vi "KI6221.vi"() -> ()   [LabVIEW 2025] (continued)
                        n2236 = Number To Engineering String(4:w3702) -> (0:w3710:string)  [unwired: 3 in]
                        n2237 = Number To Engineering String(4:w3694) -> (0:w3709:string)  [unwired: 3 in]
                        n2238 = Number To Engineering String(4:w3701) -> (0:w3723:string)  [unwired: 3 in]
                        n2239 = Number To Engineering String(4:w3722) -> (0:w3721:string)  [unwired: 3 in]
                        n2240 = Absolute Value(x=w3701) -> (abs(x)=w3719:dbl)
                        n2241 = Absolute Value(x=w3702) -> (abs(x)=w3720:dbl)
                        n2242 = local read "DAMPING"() -> (w3707:bool)
                        n2243 = local read "Voltage Measure Range"() -> (w3703:dbl)
                        n2244 = Greater?(x=w3719, y=w3720) -> (0:w3717:bool)
                        n2245 = Select(t=w3719, s=w3717, f=w3720) -> (s? t:f=w3718:dbl)
                        n2246 = Number To Exponential String(number=w3718) -> (E-format string=w3705:string)  [unwired: 3 in]
                        n2247 = Boolean To (0,1)(Boolean=w3707) -> (0, 1=w3708:i16)
                        n2248 = Number To Decimal String(number=w3700) -> (decimal integer string=w3714:string)  [unwired: 1 in]
                        n2249 = Number To Exponential String(number=w3703) -> (E-format string=w3704:string)  [unwired: 3 in]
                        n2250 = Number To Decimal String(number=w3708) -> (decimal integer string=w3706:string)  [unwired: 1 in]
                        n2251 = case shown="1" w3699 {
                          tunnel: w3714 -> [w3732 w3736 w3739]
                          tunnel: [w3732 w3736 w3739] -> w3711
                          tunnel: ["MOV" "MOV" "REP"] -> w3713
                          tunnel: ["0" "1" "1"] -> w3712
                          frame 0, Default {
                          }
                          frame 1 {
                          }
                          frame 2 {
                          }
                        }
                        n2252 = Insert Into Array(array=string[] [], new element #1=w3724, new element #2=w3723, new element #3=w3721, new element #4=w3704, new element #5=w3715, new element #6=w3713, new element #7=w3712, new element #8=w3711, new element #9=w3710, new element #10=w3709, new element #11=w3706, new element #12=w3705) -> (w3726:string[])  [unwired: 1 in]
                        n2253 = call "VisaVarReplace.vi"("Replace Array"=w3726, "Search Array"=string[] ["<DEMOSETUPSTRING>", "<DEMOSOURCE>", "<DEMOCOMP>", "<DEMORANGE>", "<DEMODELTANPLC>", "<DEMOFTYPE>", "<DEMOFSTATE>", "<DEMOFCOUNT>", "<DELTALOW>", "<DELTADELAY>", "<DELTADAMPING>", "<DELTACURRRANGE>"], "GPIB Array"=w3729) -> ("GPIB Array OUT"=w3728:string[])
                        n2254 = call "DeltaModeDemo.vi"("6220 VISA Ref"=w3730, "GPIB ARRAY"=w3728, "Current HI"=w3698, "Current LO"=w3697) -> ()  [unwired: 12 in]
                      }
                    }
                  }
                }
                n2255 = case shown="True" "CLEAR DELTA DATA" {
                  frame False {
                  }
                  frame True {
                    n2256 = invoke on="Delta Mode Measurement Data" class="Table" method="Reinit To Default"() -> ()  [unwired: 3 in, 3 out]
                    n2257 = invoke on="Delta Mode Resistance Graph" class="XYGraph (strict)" method="Reinit To Default"() -> ()  [unwired: 3 in, 3 out]
                  }
                }
                n2258 = case shown="1, Default" "FILTER" {
                  tunnel: [FALSE TRUE] -> w3669
                  frame 0 {
                  }
                  frame 1, Default {
                  }
                }
                n2259 = property on="Filter\nCount" class="DigNum (strict)"("Visible"=w3669) -> ()  [unwired: 2 in, 2 out]
                n2260 = case shown="True" "SAVE DELTA DATA" {
                  frame False {
                  }
                  frame True {
                    n2261 = File Dialog(4:"KI Data files" ("pattern label"), 5:"Save As" ("button label"), 6:"*.kdf" ("pattern label")) -> (1:w4176:bool, 3:w4175:path)  [unwired: 4 in, 2 out]
                    n2262 = case shown="False" w4176 {
                      tunnel: w4175 -> [w4180 _]
                      frame False {
                        w4184 = "%s" ("format string")
                        n2263 = property on="Delta Mode Measurement Data" class="Tbl (strict)"() -> ("Column Header Strings[]"=w4185:string[], "Value"=w4186:string[][])  [unwired: 2 in, 2 out]
                        n2264 = Array To Spreadsheet String(array=w4186, 3:w4184) -> (spreadsheet string=w4182:string)  [unwired: 1 in]
                        n2265 = Array To Spreadsheet String(array=w4185, 3:w4184) -> (spreadsheet string=w4183:string)  [unwired: 1 in]
                        n2266 = Concatenate Strings(w4183, w4182) -> (w4181:string)
                        n2267 = call "WriteToFile.vi"("character string"=w4181, "file path (dialog if empty)"=w4180) -> ()  [unwired: 3 in, 1 out]
                      }
                      frame True {
                      }
                    }
                  }
                }
                n2268 = Boolean To (0,1)(Boolean="INFINITE DELTA CYCLES") -> (0, 1=w3667:i16)
                n2269 = Multiply(x=w3667, y=i16 2) -> (x*y=w3666:i16)
                n2270 = property on="Number of cycles" class="DigNum (strict)"("Disabled"=w3666) -> ()  [unwired: 2 in, 2 out]
                n2271 = local read "Delta Mode Measurement Data"() -> (w3649:string[][])
                n2272 = local read "X AXIS LAST -DELTA"() -> (w3647:i32)
                n2273 = local read "Y AXIS LAST -DELTA"() -> (w3646:i32)
                n2274 = property on="X Axis:" class="Ring (strict)"() -> ("Value"=w3659:u16, "Strings []"=w3657:string[])  [unwired: 2 in, 2 out]
                n2275 = property on="Y Axis:" class="Ring (strict)"() -> ("Value"=w3658:u16, "Strings []"=w3656:string[])  [unwired: 2 in, 2 out]
                n2276 = Array Size(array=w3649) -> (size(s)=w3655:i32[])
                n2277 = Equal?(x=w3646, y=w3658) -> (x = y?=w3662:bool)
                n2278 = Index Array(array=w3655) -> (element=w3653:i32)  [unwired: 1 in]
                n2279 = Index Array(array=w3655) -> (element=w3654:i32)  [unwired: 1 in]
                n2280 = Equal?(x=w3647, y=w3659) -> (x = y?=w3661:bool)
                n2281 = And(x=w3661, y=w3662) -> (x .and. y?=w3660:bool)
                n2282 = Add(x=w3654, y=w3653) -> (x+y=w3652:i32)
                n2283 = Equal To 0?(x=w3652) -> (x = 0?=w3650:bool)
                n2284 = Or(x=w3660, y=w3650) -> (x .or. y?=w3651:bool)
                n2285 = case shown="False" w3651 {
                  tunnel: w3659 -> [w3741 _]
                  tunnel: w3658 -> [w3742 _]
                  tunnel: w3657 -> [w3747 _]
                  tunnel: w3656 -> [w3746 _]
                  tunnel: w3649 -> [w3743 _]
                  frame False {
                    n2286 = Index Array(array=w3747, index=w3741) -> (element=w3745:string)
                    n2287 = Index Array(array=w3746, index=w3742) -> (element=w3744:string)
                    n2288 = Add(x=w3742, y=2) -> (x+y=w3748:i32)
                    n2289 = property on="Delta Mode Resistance Graph" class="XYGraph (strict)"("X Scale.Name Label.Text"=w3745, "Y Scale.Name Label.Text"=w3744) -> ()  [unwired: 2 in, 2 out]
                    n2290 = Index Array(array=w3743, index (col)=w3741) -> (element=w3754:string[])  [unwired: 1 in]
                    n2291 = Index Array(array=w3743, index (col)=w3748) -> (element=w3751:string[])  [unwired: 1 in]
                    n2292 = Fract/Exp String To Number(string=w3754) -> (number=w3753:dbl[])  [unwired: 3 in, 1 out]
                    n2293 = Fract/Exp String To Number(string=w3751) -> (number=w3750:dbl[])  [unwired: 3 in, 1 out]
                    n2294 = call "Convert to Dynamic Data7"("Array"=w3753) -> ("Dynamic Data Type"=w3752:dynamicdata)  [unwired: 3 in]
                    n2295 = call "Convert to Dynamic Data8"("Array"=w3750) -> ("Dynamic Data Type"=w3749:dynamicdata)  [unwired: 3 in]
                    n2296 = call "Build XY Graph5"("Y Input"=w3749, "X Input"=w3752) -> ("XY Graph"=→"Delta Mode Resistance Graph":cluster{"Y":dbl[], "Y":dbl[]}[])  [unwired: 8 in, 1 out]
                    "Y AXIS LAST -DELTA" <- w3742
                    "X AXIS LAST -DELTA" <- w3741
                  }
                  frame True {
                  }
                }
              }
              frame "ARB Waveform Generator" {
                # "TURNS OFF SCALAR WHEN ITEM IS SELECTED IN CALC WINDOW 2"
                # "This inserts waves selected on\n the scratchpad into the \nComplete waveform."
                # "This deletes the highlighted \nwave from the scratchpad."
                # "ADD to the SCRATCHPAD. Whenever possible Labview signal generator subvis are used. \nElse they the signal is created in while loops."
                # "This saves the complete wave to a TEXT FILE."
                # "Updates the GRAPH\npreview based on \nthe view and \nselection settings."
                # "Update enable state based \non checkbox."
                # "Updates the tabs to match \nthe RING."
                # "These below are the segments for the GUI response to changes in the RING & Checkbox Controls."
                # "This section runs the ARB upload, run, and stop buttons. This \nsends all the information to the instrument for these buttons."
                # "Takes a complete wave and compacts it into\none wave on the scratchpad."
                # "These are controls referenced, but not directly used\nin the ARB."
                # "This is the option in the case statement for the ARB Waveform Generator. The buttons are attached to case statements that function only when the button is pressed."
                # "PHASE SETUP window. Sets the state, triggerline, and angle \n                                for the Phase marker."
                n2297 = Equal?(x=u16 4, y="Waveform Type") -> (x = y?=w4202:bool)
                n2298 = Equal?(x="Custom points file:", y=path "") -> (x = y?=w4203:bool)
                n2299 = And(x=w4203, y=w4202) -> (x .and. y?=w4199:bool)
                n2300 = Not(x=w4199) -> (.not. x?=w4198:bool)
                n2301 = And(x="ADD SCRATCH", y=w4198) -> (x .and. y?=w4200:bool)
                n2302 = case shown="True" "<- Compact" {
                  tunnel: "waveform holder" -> [_ w4280]
                  frame False {
                  }
                  frame True {
                    n2303 = control-ref of="ScratchPad"() -> (w4288:refnum<vi>)
                    n2304 = control-ref of="Complete Waveform"() -> (w4284:refnum<vi>)
                    n2305 = control-ref of="ADD"() -> (w4283:refnum<vi>)
                    n2306 = control-ref of="ADD 2"() -> (w4282:refnum<vi>)
                    n2307 = control-ref of="filter"() -> (w4281:refnum<vi>)
                    n2308 = control-ref of="ScratchPad Array"() -> (w4287:refnum<vi>)
                    n2309 = control-ref of="ScratchPad Array Cnt"() -> (w4286:refnum<vi>)
                    n2310 = control-ref of="empty"() -> (w4285:refnum<vi>)
                    n2311 = call "WaveCompact.vi"("reference"=w4288, "waveform holder"=w4280, "reference 2"=w4287, "reference 3"=w4286, "reference 5"=w4284, "reference 4"=w4285, "reference 8"=w4281, "reference 7"=w4282, "reference 6"=w4283) -> ()
                  }
                }
                n2312 = case shown="True" "Save to File" {
                  tunnel: "waveform holder" -> [_ w4297]
                  frame False {
                  }
                  frame True {
                    n2313 = property on="Complete Waveform" class="LstBox (strict)"() -> ("Item Names"=w4301:string[])  [unwired: 2 in, 2 out]
                    n2314 = Index Array(array=w4301, index=0) -> (element=w4300:string)
                    n2315 = Equal?(x=w4300, y="") -> (x = y?=w4298:bool)
                    n2316 = case shown="False" w4298 {
                      tunnel: w4297 -> [w4305 _]
                      frame False {
                        n2317 = File Dialog(4:"data.txt", 6:"*.txt") -> (1:w4307:bool, 3:w4306:path)  [unwired: 5 in, 2 out]
                        n2318 = case shown="False" w4307 {
                          tunnel: w4305 -> [w4311 _]
                          tunnel: w4306 -> [w4309 _]
                          frame False {
                            n2319 = call-poly <vilib>:"Write To Spreadsheet File.vi"("transpose? (no:F)"=TRUE, "format (%.3f)"="%.6e", "1D data"=w4311, "file path (dialog if empty)"=w4309) -> ()  [unwired: 4 in, 1 out]
                          }
                          frame True {
                          }
                        }
                      }
                      frame True {
                        n2320 = call "Display Message to User17"() -> ()  [unwired: 10 in, 2 out]
                      }
                    }
                  }
                }
                n2321 = case shown="True" w4200 {
                  tunnel: "Waveform Type" -> [_ w4367]
                  tunnel: "Custom points file:" -> [_ w4369]
                  frame False {
                  }
                  frame True {
                    n2322 = Increment(x="Rise/Fall in points") -> (x+1=w4335:i32)
                    n2323 = property on="ADD SCRATCH" class="Bool"("Disabled"=2 ("index")) -> (error out=w4340:errorcluster)  [unwired: 2 in, 1 out]
                    n2324 = property on="ScratchPad" class="LstBox (strict)"() -> ("Item Names"=w4374:string[])  [unwired: 2 in, 2 out]
                    n2325 = call "WaveErrorFlags.vi"("Rise/Fall in points"=w4335, "Number of Points per cycle"="Number of Points per cycle", "Waveform Type"=w4367, "Item Names"=w4374) -> ("Boolean 2"=w4371:bool, "Boolean 5"=w4375:bool, "Boolean 4"=w4373:bool, "Boolean"=w4370:bool, "Boolean 3"=w4372:bool)
                    n2326 = case shown="False" w4375 {
                      tunnel: w4373 -> [_ w4495]
                      tunnel: w4372 -> [_ w4494]
                      tunnel: w4371 -> [_ w4493]
                      tunnel: w4370 -> [_ w4492]
                      tunnel: w4369 -> [w4416 _]
                      tunnel: w4367 -> [w4415 _]
                      tunnel: "Analog filter - \nTau in # points" -> [w4414 _]
                      tunnel: "ADD" -> [w4413 _]
                      tunnel: "math" -> [w4412 _]
                      tunnel: "ADD 2" -> [w4411 _]
                      tunnel: "Number of Points per cycle" -> [w4410 _]
                      tunnel: "Number of Cycles" -> [w4409 _]
                      tunnel: "Standard Deviation" -> [w4408 _]
                      tunnel: "Offset (Amps)" -> [w4407 _]
                      tunnel: "Number of Points per cycle" -> [w4406 _]
                      tunnel: "Number of Cycles" -> [w4405 _]
                      tunnel: "Amplitude (Amps)" -> [w4404 _]
                      tunnel: "Offset (Amps)" -> [w4403 _]
                      tunnel: "Start Phase \n(Degrees)" -> [w4402 _]
                      tunnel: w4335 -> [w4401 _]
                      tunnel: "Number of Points per cycle" -> [w4400 _]
                      tunnel: "Number of Cycles" -> [w4399 _]
                      tunnel: "Amplitude (Amps)" -> [w4398 _]
                      tunnel: "Offset (Amps)" -> [w4397 _]
                      tunnel: "Start Phase \n(Degrees)" -> [w4396 _]
                      tunnel: "Duty Cycle (%)" -> [w4395 _]
                      tunnel: "Ramp to: (Amps)" -> [w4394 _]
                      tunnel: "Ramp from: (Amps)" -> [w4393 _]
                      tunnel: "Duty Cycle (%)" -> [w4392 _]
                      tunnel: "Start Phase \n(Degrees)" -> [w4391 _]
                      tunnel: "Number of Points per cycle" -> [w4390 _]
                      tunnel: "Number of Cycles" -> [w4389 _]
                      tunnel: w4340 -> [w4388 w4491]
                      tunnel: [w4388 w4491] -> w4338
                      tunnel: "Scalar?" -> [w4377 _]
                      tunnel: "Constant" -> [w4376 _]
                      frame False {
                        n2327 = property on="ScratchPad Array" class="Arr (strict)"() -> ("Value"=w4417:dbl[][])  [unwired: 2 in, 2 out]
                        n2328 = property on="ScratchPad Array Cnt" class="Arr (strict)"() -> ("Value"=w4418:i32[])  [unwired: 2 in, 2 out]
                        n2329 = property on="empty" class="Arr (strict)"() -> ("Value"=w4420:dbl[])  [unwired: 2 in, 2 out]
                        n2330 = case shown="1" w4415 {
                          tunnel: [w4429 w4441 w4451 w4460 w4466 w4476 w4484] -> w4422
                          tunnel: [w4433 w4444 w4454 w4463 w4470 w4477 w4486] -> w4419
                          tunnel: [w4432 w4445 w4455 w4464 errorcluster {"status"=FALSE, "code"=0, "source"=""} ("error out 9") errorcluster {"status"=FALSE, "code"=0, "source"=""} errorcluster {"status"=FALSE, "code"=0, "source"=""}] -> w4378
                          tunnel: [w4431 w4443 w4453 w4462 w4468 w4478 w4483] -> w4421
                          tunnel: w4420 -> [w4430 w4442 w4452 w4461 w4467 _ _]
                          tunnel: w4418 -> [_ _ _ _ _ w4480 w4489]
                          tunnel: w4417 -> [_ _ _ _ _ w4481 w4488]
                          tunnel: w4416 -> [_ _ _ _ w4465 _ _]
                          tunnel: w4414 -> [_ _ _ _ _ _ w4482]
                          tunnel: w4413 -> [_ _ _ _ _ w4475 _]
                          tunnel: w4412 -> [_ _ _ _ _ w4474 _]
                          tunnel: w4411 -> [_ _ _ _ _ w4473 _]
                          tunnel: w4410 -> [_ _ _ w4459 _ _ _]
                          tunnel: w4409 -> [_ _ _ w4458 _ _ _]
                          tunnel: w4408 -> [_ _ _ w4457 _ _ _]
                          tunnel: w4407 -> [_ _ _ w4456 _ _ _]
                          tunnel: w4406 -> [_ _ w4450 _ _ _ _]
                          tunnel: w4405 -> [_ _ w4449 _ _ _ _]
                          tunnel: w4404 -> [_ _ w4448 _ _ _ _]
                          tunnel: w4403 -> [_ _ w4447 _ _ _ _]
                          tunnel: w4402 -> [_ _ w4446 _ _ _ _]
                          tunnel: w4401 -> [_ w4440 _ _ _ _ _]
                          tunnel: w4400 -> [_ w4439 _ _ _ _ _]
                          tunnel: w4399 -> [_ w4438 _ _ _ _ _]
                          tunnel: w4398 -> [_ w4437 _ _ _ _ _]
                          tunnel: w4397 -> [_ w4436 _ _ _ _ _]
                          tunnel: w4396 -> [_ w4435 _ _ _ _ _]
                          tunnel: w4395 -> [_ w4434 _ _ _ _ _]
                          tunnel: w4394 -> [w4428 _ _ _ _ _ _]
                          tunnel: w4393 -> [w4427 _ _ _ _ _ _]
                          tunnel: w4392 -> [w4426 _ _ _ _ _ _]
                          tunnel: w4391 -> [w4425 _ _ _ _ _ _]
                          tunnel: w4390 -> [w4424 _ _ _ _ _ _]
                          tunnel: w4389 -> [w4423 _ _ _ _ _ _]
                          tunnel: w4377 -> [_ _ _ _ _ w4472 _]
                          tunnel: w4376 -> [_ _ _ _ _ w4471 _]
                          frame 0, Default {
                            n2331 = call "RampGen.vi"("Value 2"=w4430, "Ramp to: (Amps)"=w4428, "Ramp from: (Amps)"=w4427, "Number of Cycles"=w4423, "Duty Cycle (%)"=w4426, "Number of Points per cycle"=w4424, "Start Phase \n(Degrees)"=w4425) -> ("error"=w4432:errorcluster, "Numeric"=w4431:dbl, "String"=w4433:string, "Value"=w4429:dbl[])
                          }
                          frame 1 {
                            n2332 = call "SquareGen.vi"("Amplitude (Amps)"=w4437, "Number of Points per cycle"=w4439, "Number of Cycles"=w4438, "Value 2"=w4442, "Duty Cycle (%)"=w4434, "Offset (Amps)"=w4436, "Rise/Fall in points"=w4440, "Start Phase \n(Degrees)"=w4435) -> ("error"=w4445:errorcluster, "Numeric"=w4443:dbl, "String"=w4444:string, "Value"=w4441:dbl[])
                          }
                          frame 2 {
                            n2333 = call "SineGen.vi"("Start Phase \n(Degrees)"=w4446, "Value 2"=w4452, "Offset (Amps)"=w4447, "Amplitude (Amps)"=w4448, "Number of Points per cycle"=w4450, "Number of Cycles"=w4449) -> ("error"=w4455:errorcluster, "Numeric"=w4453:dbl, "String"=w4454:string, "Value"=w4451:dbl[])
                          }
                          frame 3 {
                            n2334 = call "NoiseGen.vi"("Offset (Amps)"=w4456, "Number of Cycles"=w4458, "Standard Deviation"=w4457, "Number of Points per cycle"=w4459, "Value 2"=w4461) -> ("error out 9"=w4464:errorcluster, "Numeric"=w4462:dbl, "String"=w4463:string, "Value"=w4460:dbl[])
                          }
                          frame 4 {
                            n2335 = call "CustomGen.vi"("Custom points file:"=w4465, "Value 2"=w4467) -> ("Value"=w4466:dbl[], "source"=w4470:string, "Numeric"=w4468:dbl)
                          }
                          frame 5 {
                            n2336 = call "CalcGen.vi"("Constant"=w4471, "Scalar?"=w4472, "Value 2"=w4480, "Value 3"=w4481, "ADD 2"=w4473, "ADD"=w4475, "math"=w4474) -> ("Numeric"=w4478:dbl, "source"=w4477:string, "Value"=w4476:dbl[])
                          }
                          frame 6 {
                            n2337 = call "FilterGen.vi"("SP ARRAY"=w4488, "Analog filter - \nTau in # points"=w4482, "Value 3"=w4489, "filter"="filter") -> ("Numeric"=w4483:dbl, "source"=w4486:string, "Value"=w4484:dbl[])
                          }
                        }
                        "error out 9" <- w4378
                        n2338 = control-ref of="ScratchPad"() -> (w4387:refnum<vi>)
                        n2339 = control-ref of="Complete Waveform"() -> (w4384:refnum<vi>)
                        n2340 = control-ref of="ADD"() -> (w4383:refnum<vi>)
                        n2341 = control-ref of="ADD 2"() -> (w4382:refnum<vi>)
                        n2342 = control-ref of="filter"() -> (w4381:refnum<vi>)
                        n2343 = control-ref of="Pad Last"() -> (w4380:refnum<vi>)
                        n2344 = control-ref of="Graph Last"() -> (w4379:refnum<vi>)
                        n2345 = control-ref of="ScratchPad Array"() -> (w4386:refnum<vi>)
                        n2346 = control-ref of="ScratchPad Array Cnt"() -> (w4385:refnum<vi>)
                        n2347 = call "AddWaveToPad.vi"("Filter"=w4381, "Pad LAST"=w4380, "Graph LAST"=w4379, "Value"=w4422, "Add 2"=w4382, "Numeric"=w4421, "Add"=w4383, "String"=w4419, "Complete Waveform"=w4384, "ScratchPad Array Count"=w4385, "ScratchPad Array"=w4386, "ScratchPad"=w4387) -> ()
                      }
                      frame True {
                        n2348 = control-ref of="Rise/Fall in points"() -> (w4490:refnum<vi>)
                        n2349 = call "WaveAddErrors.vi"("Boolean 2"=w4493, "Boolean 3"=w4494, "Boolean"=w4492, "Boolean 4"=w4495, "reference"=w4490) -> ()
                      }
                    }
                    n2350 = property on="ADD SCRATCH" class="Bool"(error in=w4338, "Disabled"=0 ("index")) -> ()  [unwired: 1 in, 2 out]
                  }
                }
                n2351 = local read "DEMO MODE"() -> (w4197:bool)
                n2352 = Compound Arithmetic op=OR("RUN", "STOP", "UPLOAD") -> (w4205:bool)
                n2353 = And(x=w4197, y=w4205) -> (x .and. y?=w4206:bool)
                n2354 = Not(x=w4197) -> (.not. x?=w4207:bool)
                n2355 = And(x=w4205, y=w4207) -> (x .and. y?=w4208:bool)
                n2356 = case shown="True" w4208 {
                  tunnel: "RUN" -> [_ w4253]
                  tunnel: "STOP" -> [_ w4254]
                  tunnel: "UPLOAD" -> [_ w4252]
                  tunnel: w4206 -> [w4234 _]
                  frame False {
                    n2357 = call "Demo Mode"("Enable"=w4234) -> ()  [unwired: 9 in, 2 out]
                  }
                  frame True {
                    n2358 = control-ref of="6220 VISA"() -> (w4250:refnum<vi>)
                    n2359 = control-ref of="Setup String"() -> (w4237:refnum<vi>)
                    n2360 = control-ref of="UPLOAD TIME WINDOW"() -> (w4249:refnum<vi>)
                    n2361 = control-ref of="triggerline"() -> (w4246:refnum<vi>)
                    n2362 = control-ref of="INF"() -> (w4248:refnum<vi>)
                    n2363 = control-ref of="STOP"() -> (w4244:refnum<vi>)
                    n2364 = control-ref of="phase enable"() -> (w4245:refnum<vi>)
                    n2365 = control-ref of="RUN"() -> (w4243:refnum<vi>)
                    n2366 = control-ref of="UPLOAD"() -> (w4242:refnum<vi>)
                    n2367 = control-ref of="Phase Value"() -> (w4247:refnum<vi>)
                    n2368 = control-ref of="GPIB Array"() -> (w4240:refnum<vi>)
                    n2369 = control-ref of="waveform holder"() -> (w4241:refnum<vi>)
                    n2370 = call "ArbVisa.vi"("Waveform Holder"=w4241, "SETUPSTRING"=w4237, "Run Button"=w4243, "Stop Button"=w4244, "Phase Value (angle)"=w4247, "GPIB ARRAY"=w4240, "UPLOAD"=w4252, "Upload Button"=w4242, "Total Wave Duration (S)"="Total Wave Duration (S)", "INF duration"=w4248, "Signal Repetition \nFrequency (Hz)"="Signal Repetition \nFrequency (Hz)", "Upload Window"=w4249, "Voltage\n Compliance"="Voltage\n Compliance", "Triggerline"=w4246, "Last Amplitude sent"="last amp", "RUN"=w4253, "STOP"=w4254, "Phase Enable State"=w4245, "6220 VISA"=w4250) -> ("Last Amplitude sent 2"=w4235:string)
                    n2371 = local write "last amp"(w4235) -> ()
                  }
                }
                n2372 = case shown="True" "phaseMarker Setup" {
                  frame False {
                  }
                  frame True {
                    n2373 = property on="Phase Value" class="DigNum (strict)"() -> ("Value"=w4256:dbl)  [unwired: 2 in, 2 out]
                    n2374 = property on="triggerline" class="DigNum (strict)"() -> ("Value"=w4257:i16)  [unwired: 2 in, 2 out]
                    n2375 = property on="phase enable" class="Bool (strict)"() -> ("Value"=w4255:bool)  [unwired: 2 in, 2 out]
                    n2376 = call "phasesubvi2.vi"("Phase value (degrees)"=w4256, "Triggerline"=w4257, "Enable Phase Marker"=w4255) -> ("Enable Phase Marker 2"=w4258:bool, "Phase value"=w4261:dbl, "Triggerline 2"=w4260:i16, "OK"=w4259:bool)  [unwired: 19 in, 2 out]
                    n2377 = case shown="True" w4259 {
                      tunnel: w4258 -> [_ w4264]
                      tunnel: w4261 -> [_ w4263]
                      tunnel: w4260 -> [_ w4262]
                      frame False {
                      }
                      frame True {
                        "phase enable" <- w4264
                        "Phase Value" <- w4263
                        "triggerline" <- w4262
                      }
                    }
                  }
                }
                n2378 = case shown="True" "DELETE SCRATCH" {
                  frame False {
                  }
                  frame True {
                    n2379 = control-ref of="ScratchPad Array"() -> (w4333:refnum<vi>)
                    n2380 = control-ref of="ScratchPad"() -> (w4334:refnum<vi>)
                    n2381 = control-ref of="ADD"() -> (w4330:refnum<vi>)
                    n2382 = control-ref of="filter"() -> (w4331:refnum<vi>)
                    n2383 = control-ref of="ScratchPad Array Cnt"() -> (w4332:refnum<vi>)
                    n2384 = control-ref of="ADD 2"() -> (w4329:refnum<vi>)
                    n2385 = control-ref of="Graph Last"() -> (w4328:refnum<vi>)
                    n2386 = control-ref of="Pad Last"() -> (w4327:refnum<vi>)
                    n2387 = call "DeleteWave.vi"("ADD 2"=w4329, "Graph Last"=w4328, "ADD"=w4330, "Pad Last"=w4327, "Filter"=w4331, "ScratchPad Array Cnt"=w4332, "ScratchPad Array"=w4333, "Scratchpad"=w4334) -> ()
                  }
                }
                n2388 = Boolean To (0,1)(Boolean="INF") -> (0, 1=w4224:i16)
                n2389 = property on="Waveform Type" class="Ring (strict)"() -> ("Value"=w4230:u16)  [unwired: 2 in, 2 out]
                n2390 = Multiply(x=w4224, y=i16 2) -> (x*y=w4223:i16)
                n2391 = property on="Total Wave Duration (S)" class="DigNum (strict)"("Disabled"=w4223) -> ()  [unwired: 2 in, 2 out]
                n2392 = property on="waveform tabs" class="TabCtl (strict)"("Value"=w4230) -> ()  [unwired: 2 in, 2 out]
                n2393 = local read "Graph Last"() -> (w4195:i32)
                n2394 = local read "Pad Last"() -> (w4196:i32)
                n2395 = Index Array(array="ScratchPad", index=0) -> (element=w4215:i32)
                n2396 = Not Equal?(x=w4215, y=w4196) -> (x != y?=w4216:bool)
                n2397 = Not Equal?(x="Graph view:", y=w4195) -> (x != y?=w4218:bool)
                n2398 = case shown="True" w4216 {
                  tunnel: w4215 -> [_ w4270]
                  tunnel: "Graph view:" -> [_ w4269]
                  tunnel: [w4265 w4266] -> w4213
                  frame False {
                    n2399 = local read "selection"() -> (w4265:dbl[])
                  }
                  frame True {
                    n2400 = local read "ScratchPad Array Cnt"() -> (w4267:i32[])
                    n2401 = local read "ScratchPad Array"() -> (w4268:dbl[][])
                    n2402 = Index Array(array=w4268, index (row)=w4270) -> (element=w4272:dbl[])  [unwired: 1 in]
                    n2403 = Index Array(array=w4267, index=w4270) -> (element=w4271:i32)
                    n2404 = Array Subset(array=w4272, length=w4271) -> (w4266:dbl[])  [unwired: 1 in]
                    "selection" <- w4266
                    n2405 = case shown="0, Default" w4269 {
                      tunnel: w4266 -> [_ w4273]
                      frame 0, Default {
                      }
                      frame 1 {
                        n2406 = local write "Waveform\n Preview"(w4273) -> ()
                      }
                    }
                    "Pad Last" <- w4270
                  }
                }
                n2407 = case shown="True" w4218 {
                  tunnel: "Graph view:" -> [_ w4277]
                  tunnel: w4213 -> [_ w4276]
                  tunnel: "waveform holder" -> [_ w4274]
                  frame False {
                  }
                  frame True {
                    n2408 = case shown="0, Default" w4277 {
                      tunnel: [w4278 w4279] -> w4275
                      tunnel: w4276 -> [_ w4279]
                      tunnel: w4274 -> [w4278 _]
                      frame 0, Default {
                      }
                      frame 1 {
                      }
                    }
                    "Waveform\n Preview" <- w4275
                    "Graph Last" <- w4277
                  }
                }
                n2409 = case shown="True" "rename" {
                  frame False {
                  }
                  frame True {
                    # "This is the code to \nrename a wave on\nthe scratchpad..."
                    n2410 = property on="ScratchPad" class="LstBox (strict)"() -> (error out=w4296:errorcluster, "Item Names"=w4292:string[], "Value"=w4295:i32[])  [unwired: 2 in, 1 out]
                    n2411 = Index Array(array=w4295, index=0) -> (element=w4291:i32)
                    n2412 = Index Array(array=w4292, index=w4291) -> (element=w4290:string)
                    n2413 = call "renameWindow.vi"("Waveform Name IN"=w4290) -> ("Waveform Name OUT"=w4289:string)
                    n2414 = Replace Array Subset(array=w4292, new element=w4289, index=w4291) -> (w4293:string[])
                    n2415 = property on="ADD 2" class="LstBox (strict)"("Item Names"=w4293) -> ()  [unwired: 2 in, 2 out]
                    n2416 = property on="ADD" class="LstBox (strict)"("Item Names"=w4293) -> ()  [unwired: 2 in, 2 out]
                    n2417 = property on="ScratchPad" class="LstBox (strict)"(error in=w4296, "Item Names"=w4293) -> ()  [unwired: 1 in, 2 out]
                    n2418 = property on="filter" class="LstBox (strict)"("Item Names"=w4293) -> ()  [unwired: 2 in, 2 out]
                  }
                }
                n2419 = case shown="True" "DELETE COMPLETE" {
                  frame False {
                  }
                  frame True {
                    n2420 = control-ref of="Complete Array Cnt"() -> (w4324:refnum<vi>)
                    n2421 = control-ref of="Waveform\n Preview"() -> (w4322:refnum<vi>)
                    n2422 = control-ref of="Graph view:"() -> (w4323:refnum<vi>)
                    n2423 = control-ref of="waveform holder"() -> (w4321:refnum<vi>)
                    n2424 = control-ref of="Complete Waveform"() -> (w4326:refnum<vi>)
                    n2425 = control-ref of="Complete Array"() -> (w4325:refnum<vi>)
                    n2426 = call "DeleteCompWave.vi"("reference"=w4326, "reference 6"=w4321, "reference 2"=w4325, "reference 3"=w4324, "reference 4"=w4323, "reference 5"=w4322) -> ()
                  }
                }
                n2427 = property on="ADD 2" class="LstBox (strict)"() -> ("Key Focus"=w4190:bool)  [unwired: 2 in, 2 out]
                n2428 = case shown="True" "ADD COMPLETE" {
                  tunnel: "Graph view:" -> [_ w4320]
                  frame False {
                  }
                  frame True {
                    n2429 = control-ref of="Waveform\n Preview"() -> (w4312:refnum<vi>)
                    n2430 = control-ref of="ScratchPad"() -> (w4319:refnum<vi>)
                    n2431 = control-ref of="Complete Waveform"() -> (w4317:refnum<vi>)
                    n2432 = control-ref of="ScratchPad Array"() -> (w4318:refnum<vi>)
                    n2433 = control-ref of="Complete Array"() -> (w4316:refnum<vi>)
                    n2434 = control-ref of="waveform holder"() -> (w4315:refnum<vi>)
                    n2435 = control-ref of="Complete Array Cnt"() -> (w4314:refnum<vi>)
                    n2436 = control-ref of="ScratchPad Array Cnt"() -> (w4313:refnum<vi>)
                    n2437 = call "AddCompWave.vi"("reference"=w4319, "Graph view:"=w4320, "reference 2"=w4318, "reference 3"=w4317, "reference 5"=w4315, "reference 4"=w4316, "reference 8"=w4312, "reference 7"=w4313, "reference 6"=w4314) -> ()
                  }
                }
                n2438 = case shown="True" w4190 {
                  frame False {
                  }
                  frame True {
                    n2439 = local write "Scalar?"(FALSE ("Scalar?")) -> ()
                  }
                }
                n2440 = case shown="True" "ARB HELP LINK" {
                  frame False {
                  }
                  frame True {
                    n2441 = call "DecideWindow.vi"("INDEX"=7, "wizard?"=0) -> ()  [unwired: 9 in, 5 out]
                  }
                }
              }
            }
          }
          frame "Front Panel" {
            # "This cover protects the \nbuttons from latching until \ncontrol is activated."
            # "BUTTON MASK"
            n2442 = property on="Control watch" class="Bool (strict)"("Value"="CONTROL") -> ("Value"=w4497:bool)  [unwired: 2 in, 2 out]
            n2443 = local read "DEMO MODE"() -> (w4498:bool)
            n2444 = Not(x="CONTROL") -> (.not. x?=w4506:bool)
            n2445 = property on="______________________________________________________________________________________________________________" class="Bool (strict)"("Visible"=w4506) -> ()  [unwired: 2 in, 2 out]
            n2446 = local read "6220 VISA"() -> (w4500:refnum<visa-resource-name>)
            n2447 = local read "GPIB Array"() -> (w4499:string[])
            n2448 = Not(x=w4498) -> (.not. x?=w4501:bool)
            n2449 = Not Equal?(x=w4497, y="CONTROL") -> (x != y?=w4509:bool)
            n2450 = And(x=w4509, y="CONTROL") -> (x .and. y?=w4507:bool)
            n2451 = And(x=w4507, y=w4501) -> (x .and. y?=w4502:bool)
            n2452 = case shown="True" w4502 {
              tunnel: w4499 -> [_ w4521]
              tunnel: w4500 -> [_ w4520]
              tunnel: [TRUE w4519] -> w4508
              tunnel: [FALSE w4518] -> w4505
              frame False {
              }
              frame True {
                n2453 = control-ref of="FRONT PANEL 6220"() -> (w4512:refnum<vi>)
                n2454 = control-ref of="CURSOR RIGHT"() -> (w4515:refnum<vi>)
                n2455 = control-ref of="CURSOR LEFT"() -> (w4516:refnum<vi>)
                n2456 = control-ref of="knob push"() -> (w4514:refnum<vi>)
                n2457 = control-ref of="Knob"() -> (w4517:refnum<vi>)
                n2458 = call "VFPModelTest.vi"("6220 VISA"=w4520, "Knob Push"=w4514, "GPIB Array"=w4521, "Cursor Right"=w4515, "Cursor Left"=w4516, "Knob"=w4517, "6220 pic"=w4512) -> ("error out 21"=→"error out 21":errorcluster, "Boolean"=w4518:bool, "Boolean 2"=w4519:bool)
              }
            }
            n2459 = And(x="CONTROL", y=w4508) -> (x .and. y?=w4504:bool)
            n2460 = And(x=w4501, y=w4504) -> (x .and. y?=w4503:bool)
            n2461 = case shown="True" w4503 {
              selector: w4503 -> [w4522 _]
              tunnel: w4500 -> [_ w4543]
              tunnel: w4499 -> [_ w4544]
              tunnel: "CONTROL" -> [w4525 _]
              tunnel: w4505 -> [w4524 _]
              frame False {
                n2462 = And(x=w4525, y=w4524) -> (x .and. y?=w4523:bool)
                n2463 = call "INSTR not responding"("Enable"=w4523) -> ()  [unwired: 9 in, 2 out]
                n2464 = local write "CONTROL"(w4522) -> ()
              }
              frame True {
                # "This section monitors half of the\nfront panel buttons. These latch\nand activate VISA commands in the \nsubvi."
                # "This code handles the Knob turn events\nfor the 6221."
                # "The send SCPI Button code segment"
                # "The RESET button code segment"
                # "Sets delay time (button monitor interval)"
                # "These controls are referenced, but not\ndirectly used..."
                # "This section monitors half of the\nfront panel buttons. These latch\nand activate VISA commands in the \nsubvi."
                # "This code updates the Virtual display and \nsource indicator light"
                n2465 = control-ref of="LIGHT"() -> (w4539:refnum<vi>)
                n2466 = control-ref of="LITTLE DISP OVERLAY"() -> (w4538:refnum<vi>)
                n2467 = control-ref of="BIG DISP OVERLAY"() -> (w4537:refnum<vi>)
                n2468 = control-ref of="BIG DISP Ohm Overlay"() -> (w4526:refnum<vi>)
                n2469 = call "DispUpdate.vi"("Big Display Overlay"=w4537, "Value"=w4544, "Little Display Overlay"=w4538, "Light indicator"=w4539, "Big Display Ohms"=w4526, "Value 2"=w4543) -> ("error out 16"=w4540:errorcluster, "error out 15"=→"error out 15":errorcluster, "SUB READING 6220"=→"SUB READING 6220":string, "MAIN 6220 READING"=→"MAIN 6220 READING":string, "LIGHT"=→"LIGHT":bool)
                n2470 = call "VFPButtons.vi"("6220 VISA"=w4543, "DELTA"="DELTA", "SWP"="SWP", "GPIB Array"=w4544, "WAVE"="WAVE", "knob push"="knob push", "COMM"="COMM", "error out 16"=w4540, "NUM+/-"="NUM+/-", "local"="local", "ENTER"="ENTER", "MENU"="MENU", "TRIG"="TRIG", "config"="config", "FILTER"="FILTER 2", "AMPL"="AMPL", "PRES"="PRES", "UNITS"="UNITS", "RANGE UP"="RANGE UP", "PULSE"="PULSE", "EXIT 2"="EXIT", "RANGE AUTO"="RANGE AUTO", "CURSOR LEFT"="CURSOR LEFT", "RANGE DOWN"="RANGE DOWN") -> ("error"=w4548:errorcluster)  [unwired: 3 in]
                n2471 = control-ref of="LIGHT"() -> (w4531:refnum<vi>)
                n2472 = control-ref of="Knob Last"() -> (w4532:refnum<vi>)
                n2473 = Wait (ms)(milliseconds to wait="milliseconds to wait") -> ()  [unwired: 1 out]
                n2474 = case shown="True" "SEND COMM" {
                  tunnel: w4543 -> [_ w4589]
                  tunnel: [errorcluster {"status"=FALSE, "code"=0, "source"=""} ("error out") w4587] -> w4541
                  tunnel: errorcluster {"status"=FALSE, "code"=0, "source"=""} -> [_ w4586]
                  frame False {
                  }
                  frame True {
                    # "SEND COMM"
                    n2475 = Insert Into Array(array=string[] [], new element="Command String") -> (w4583:string[])  [unwired: 1 in]
                    n2476 = call "VISAreadWrite.vi"("error in (no error)"=w4586, "GPIB INDEX Array"=i32[] [0], "GPIB ARRAY"=w4583, "VISA REFERENCE"=w4589) -> ("error out 15"=w4587:errorcluster)  [unwired: 1 out]
                  }
                }
                n2477 = case shown="True" "RESET" {
                  tunnel: w4543 -> [_ w4595]
                  tunnel: w4544 -> [_ w4594]
                  tunnel: [errorcluster {"status"=FALSE, "code"=0, "source"=""} ("error out") w4592] -> w4547
                  tunnel: w4541 -> [_ w4591]
                  frame False {
                  }
                  frame True {
                    # "SEND *RST"
                    n2478 = call "VISAreadWrite.vi"("error in (no error)"=w4591, "GPIB INDEX Array"=i32[] [6], "GPIB ARRAY"=w4594, "VISA REFERENCE"=w4595) -> ("error out 15"=w4592:errorcluster)  [unwired: 1 out]
                  }
                }
                n2479 = call "KnobTurn.vi"("Knob Last"=w4532, "6220 VISA"=w4543, "GPIB Array"=w4544, "error 2"=w4547, "Knob"="Knob") -> ("error"=w4546:errorcluster)
                n2480 = call "VFPButtons2.vi"("LIGHT"=w4531, "6220 VISA"=w4543, "SAVE"="SAVE", "SETUP"="SETUP", "COND"="COND", "error"=w4546, "AVG"="AVG", "error 2"=w4548, "FREQ"="FREQ", "GPIB Array"=w4544, "TRIAX"="TRIAX", "DC"="DC", "CURSOR RIGHT"="CURSOR RIGHT", "DISP"="DISP", "OUTPUT"="OUTPUT", "RECALL"="RECALL", "ADDR"="ADDR") -> ("error 27"=→"error 27":errorcluster)  [unwired: 2 in]
              }
            }
          }
          frame "Help" {
          }
        }
        n2481 = local read "SAVE NOW"() -> (w191:bool)
        n2482 = case shown="False" "WEB UPDATES" {
          frame False {
          }
          frame True {
            n2483 = local write "WEB UPDATES"(FALSE ("WEB UPDATES")) -> ()
            n2484 = local read "Settings cluster"() -> (w228:T7)
            n2485 = Unbundle(w228) -> ("version"=w227:string)  [unwired: 4 out]
            n2486 = Concatenate Strings("To update this software go to http://www.keithley.com/redirects/6220/. The update will contain instructions and a number of compressed files. If there are any backward compatibility issues, they will be mentioned in the readme instructions with the update. Make sure only to install version numbers greater than your current installation. The current version number is: ", w227) -> (w230:string)
            n2487 = call "Display Message to User"("Message"=w230) -> ()  [unwired: 9 in, 2 out]
          }
        }
        n2488 = control-ref of="WEB UPDATE STR"() -> (w170:refnum<vi>)
        n2489 = control-ref of="Default path"() -> (w172:refnum<vi>)
        n2490 = control-ref of="WEB UPDATES"() -> (w171:refnum<vi>)
        n2491 = control-ref of="Settings cluster"() -> (w169:refnum<vi>)
        n2492 = Or(x="SAVE 2", y=w191) -> (x .or. y?=w223:bool)
        n2493 = case shown="True" w223 {
          tunnel: w191 -> [_ w4877]
          frame False {
          }
          frame True {
            # "SAVE FILE stuff"
            n2494 = local write "EXIT NOW"(w4877) -> ()
            n2495 = local write "SAVE NOW"(FALSE) -> ()
            n2496 = local read "Current Test File:"() -> (w4875:path)
            n2497 = Path To String(path=w4875) -> (string=w4874:string)
            n2498 = File Dialog(4:"KI config files" ("pattern label"), 5:"Save As" ("button label"), 6:"*.kcf" ("pattern label"), 9:w4874) -> (1:w4879:bool, 3:w4878:path)  [unwired: 3 in, 2 out]
            n2499 = case shown="False" w4879 {
              tunnel: w4878 -> [w4969 _]
              frame False {
                # "Above creates the data files\nRight - save the correct step\nsource values to the main \ncluster file."
                n2500 = property on=".  IP#2" class="DigNum (strict)"() -> ("Value"=w5056:i32)  [unwired: 2 in, 2 out]
                n2501 = property on="LOW to EARTH" class="Bool (strict)"() -> ("Value"=w5053:bool)  [unwired: 2 in, 2 out]
                n2502 = property on="Power:" class="Ring (strict)"() -> ("Value"=w5050:u16)  [unwired: 2 in, 2 out]
                n2503 = property on=".  IP#3" class="DigNum (strict)"() -> ("Value"=w5047:i32)  [unwired: 2 in, 2 out]
                n2504 = property on=".  IP#4" class="DigNum (strict)"() -> ("Value"=w5044:i32)  [unwired: 2 in, 2 out]
                n2505 = property on="Select GPIB Board number:\n(default to zero)" class="DigNum (strict)"() -> ("Value"=w5042:i32)  [unwired: 2 in, 2 out]
                n2506 = control-ref of="attachments"() -> (w4977:refnum<vi>)
                n2507 = control-ref of="Differential Conductance Measurement Data"() -> (w4976:refnum<vi>)
                n2508 = control-ref of="PULSE DATA SHEET"() -> (w4975:refnum<vi>)
                n2509 = control-ref of="Delta Mode Measurement Data"() -> (w4974:refnum<vi>)
                n2510 = property on="Complete Waveform" class="LstBox (strict)"() -> ("Item Names"=w5012:string[], "Value"=w5011:i32[])  [unwired: 2 in, 2 out]
                n2511 = property on="ScratchPad" class="LstBox (strict)"() -> ("Item Names"=w5016:string[], "Value"=w5015:i32[])  [unwired: 2 in, 2 out]
                n2512 = property on="ARB\nVoltage\n Compliance" class="DigNum (strict)"() -> ("Value"=w4981:dbl)  [unwired: 2 in, 2 out]
                n2513 = Path To String(path=path "") -> (string=w4972:string)
                n2514 = property on="Complete Array" class="Arr (strict)"() -> ("Value"=w5014:dbl[][])  [unwired: 2 in, 2 out]
                n2515 = property on="triggerline" class="DigNum (strict)"() -> ("Value"=w4982:i16)  [unwired: 2 in, 2 out]
                n2516 = property on="Number of complete cycles" class="DigNum (strict)"() -> ("Value"=w5023:dbl)  [unwired: 2 in, 2 out]
                n2517 = local read "Current Source \nVoltage Compliance (V)"() -> (w4910:dbl)
                n2518 = local read "Current Source \nVoltage Compliance (V)"() -> (w4905:dbl)
                n2519 = property on="Select the nanovoltmeter model number:" class="Ring (strict)"() -> ("Value"=w5055:u16)  [unwired: 2 in, 2 out]
                n2520 = property on="The current source is set up for easy cabling in STANDARD CONNECTIONS mode. This \nallows for many versatile measurement setups. However, with high impedance\ndevices or with significant cable capacitance the RC product in the circuit can impact the \ninstrument's risetime for some tests. If you would like to make GUARDED CONNECTIONS\nbecause of the RC present in your test system or for any other reason select GUARDED\nCONNECTIONS below, otherwise use STANDARD CONNECTIONS." class="Ring (strict)"() -> ("Value"=w5052:u16)  [unwired: 2 in, 2 out]
                n2521 = property on="HI IMP devices?" class="Ring (strict)"() -> ("Value"=w5049:u16)  [unwired: 2 in, 2 out]
                n2522 = property on="Enable \nSTEP SOURCE" class="Bool (strict)"() -> ("Value"=w5046:bool)  [unwired: 2 in, 2 out]
                n2523 = property on="Select GPIB Address number \nof the current source:" class="DigNum (strict)"() -> ("Value"=w5043:i32)  [unwired: 2 in, 2 out]
                n2524 = property on="ADD 2" class="LstBox (strict)"() -> ("Value"=w5008:i32[])  [unwired: 2 in, 2 out]
                n2525 = local read "PULSE FILTER"() -> (w4966:u16)
                n2526 = property on="ADD" class="LstBox (strict)"() -> ("Value"=w5009:i32[])  [unwired: 2 in, 2 out]
                n2527 = local read "Measurement Integration \n(NPLCs)"() -> (w4901:dbl)
                n2528 = property on="INFINITE REPEAT PULSE CYCLES" class="Bool (strict)"() -> ("Value"=w5035:bool)  [unwired: 2 in, 2 out]
                n2529 = property on="Phase Value" class="DigNum (strict)"() -> ("Value"=w4983:dbl)  [unwired: 2 in, 2 out]
                n2530 = property on="Complete Array Cnt" class="Arr (strict)"() -> ("Value"=w5013:i32[])  [unwired: 2 in, 2 out]
                n2531 = property on="filter" class="LstBox (strict)"() -> ("Value"=w5007:i32[])  [unwired: 2 in, 2 out]
                n2532 = local write "Current Test File:"(w4969) -> ()
                n2533 = property on="Select Network Card number:\n(default to zero)" class="DigNum (strict)"() -> ("Value"=w5054:i32)  [unwired: 2 in, 2 out]
                n2534 = property on="Input instrument IP Address:" class="DigNum (strict)"() -> ("Value"=w5051:i32)  [unwired: 2 in, 2 out]
                n2535 = property on="Select the interface for the 6220/6221:" class="Ring (strict)"() -> ("Value"=w5048:u16)  [unwired: 2 in, 2 out]
                n2536 = property on="Select the current source model number:" class="Ring (strict)"() -> ("Value"=w5045:u16)  [unwired: 2 in, 2 out]
                n2537 = property on="Select step source:" class="Ring (strict)"() -> ("Value"=w5032:u16)  [unwired: 2 in, 2 out]
                n2538 = property on="MASTER DRIVER Array" class="Arr (strict)"() -> ("Value"=w5031:T9)  [unwired: 2 in, 2 out]
                n2539 = local read "Delay (settle time in sec)"() -> (w4904:dbl)
                n2540 = local read "Number of sweep points"() -> (w4907:i32)
                n2541 = local read "Voltage Measure Range"() -> (w4902:dbl)
                n2542 = property on="phase enable" class="Bool (strict)"() -> ("Value"=w4984:bool)  [unwired: 2 in, 2 out]
                n2543 = local read "Start Current (Amps)"() -> (w4909:dbl)
                n2544 = local read "Stop Current (Amps)"() -> (w4908:dbl)
                n2545 = local read "Source Level (Amps)"() -> (w4911:dbl)
                n2546 = property on="waveform holder" class="Arr (strict)"() -> ("Value"=w5010:dbl[])  [unwired: 2 in, 2 out]
                n2547 = property on="ScratchPad Array" class="Arr (strict)"() -> ("Value"=w4884:dbl[][])  [unwired: 2 in, 2 out]
                n2548 = local read "enable measure"() -> (w4903:bool)
                n2549 = property on="Number of Points per cycle" class="DigNum (strict)"() -> ("Value"=w5018:i32)  [unwired: 2 in, 2 out]
                n2550 = property on="I want to control my test in terms of:" class="Ring (strict)"() -> ("Value"=w5058:u16)  [unwired: 2 in, 2 out]
                n2551 = call "SaveStepSrc.vi"("Value 5"="Test file description and comments:", "Value 4"=w5032, "Value 3"=w5031) -> ("result string 3"=w5038:string, "result string 4"=w5039:string, "result string 5"=w5040:string, "result string 6"=w5041:string, "result string 2"=w5037:string, "result string"=w5036:string, "Value"=w5029:i32, "Value 2"=w5030:i32, "String"=w5034:string)
                n2552 = local read "Sweep Type"() -> (w4906:u16)
                n2553 = local read "Setup String"() -> (w4914:string)
                n2554 = property on="Pulse Mode:" class="Ring (strict)"() -> ("Value"=w5057:u16)  [unwired: 2 in, 2 out]
                n2555 = property on="ScratchPad Array Cnt" class="Arr (strict)"() -> ("Value"=w4887:i32[])  [unwired: 2 in, 2 out]
                n2556 = property on="Waveform Type" class="Ring (strict)"() -> ("Value"=w5022:u16)  [unwired: 2 in, 2 out]
                n2557 = property on="INF" class="Bool (strict)"() -> ("Value"=w5020:bool)  [unwired: 2 in, 2 out]
                n2558 = property on="Signal Repetition \nFrequency (Hz)" class="DigNum (strict)"() -> ("Value"=w5019:dbl)  [unwired: 2 in, 2 out]
                n2559 = local read "CAP IN"() -> (w4912:u16)
                n2560 = property on="Ramp from: (Amps)" class="DigNum (strict)"() -> ("Value"=w5017:dbl)  [unwired: 2 in, 2 out]
                n2561 = property on="Graph view:" class="Ring (strict)"() -> ("Value"=w5021:u16)  [unwired: 2 in, 2 out]
                n2562 = local read "Signal Repetition \nFrequency (Hz)"() -> (w4890:dbl)
                n2563 = Array Max & Min(array=w4887) -> (max value=w4885:i32)  [unwired: 3 out]
                n2564 = local read "I Sweep V Measure Data"() -> (w4899:string[][])
                n2565 = local read "INFINITE DELTA CYCLES"() -> (w4952:bool)
                n2566 = local read "Number of Pulse Off Measurements"() -> (w4888:i32)
                n2567 = Array Subset(array=w4884, index (col)=0 ("index"), length (col)=w4885) -> (w4883:dbl[][])  [unwired: 2 in]
                n2568 = local read "Voltage\n Compliance"() -> (w4889:dbl)
                n2569 = local read "Ramp from: (Amps)"() -> (w4898:dbl)
                n2570 = local read "Amplitude (Amps)"() -> (w4895:dbl)
                n2571 = local read "Amplitude (Amps)"() -> (w4892:dbl)
                n2572 = local read "Ramp to: (Amps)"() -> (w4897:dbl)
                n2573 = local read "Waveform Type"() -> (w4900:u16)
                n2574 = local read "Duty Cycle (%)"() -> (w4896:dbl)
                n2575 = local read "Duty Cycle (%)"() -> (w4893:dbl)
                n2576 = local read "Offset (Amps)"() -> (w4894:dbl)
                n2577 = local read "Offset (Amps)"() -> (w4891:dbl)
                n2578 = local read "FILTER"() -> (w4951:u16)
                n2579 = local read "output cluster"() -> (w4936:T10)
                n2580 = property on="Standard Deviation" class="DigNum (strict)"() -> ("Value"=w5004:dbl)  [unwired: 2 in, 2 out]
                n2581 = property on="Offset (Amps)" class="DigNum (strict)"() -> ("Value"=w5005:dbl)  [unwired: 2 in, 2 out]
                n2582 = property on="Analog filter - \nTau in # points" class="DigNum (strict)"() -> ("Value"=w5006:dbl)  [unwired: 2 in, 2 out]
                n2583 = local read "FILTER"() -> (w4913:u16)
                n2584 = property on="Number of Cycles" class="DigNum (strict)"() -> ("Value"=w4986:dbl)  [unwired: 2 in, 2 out]
                n2585 = property on="Ramp to: (Amps)" class="DigNum (strict)"() -> ("Value"=w4987:dbl)  [unwired: 2 in, 2 out]
                n2586 = property on="Duty Cycle (%)" class="DigNum (strict)"() -> ("Value"=w4988:dbl)  [unwired: 2 in, 2 out]
                n2587 = property on="Start Phase \n(Degrees)" class="DigNum (strict)"() -> ("Value"=w4989:dbl)  [unwired: 2 in, 2 out]
                n2588 = property on="Number of Points per cycle" class="DigNum (strict)"() -> ("Value"=w4990:i32)  [unwired: 2 in, 2 out]
                n2589 = property on="Number of Cycles" class="DigNum (strict)"() -> ("Value"=w4991:dbl)  [unwired: 2 in, 2 out]
                n2590 = property on="Amplitude (Amps)" class="DigNum (strict)"() -> ("Value"=w4992:dbl)  [unwired: 2 in, 2 out]
                n2591 = property on="Offset (Amps)" class="DigNum (strict)"() -> ("Value"=w4993:dbl)  [unwired: 2 in, 2 out]
                n2592 = property on="Duty Cycle (%)" class="DigNum (strict)"() -> ("Value"=w4994:dbl)  [unwired: 2 in, 2 out]
                n2593 = property on="Start Phase \n(Degrees)" class="DigNum (strict)"() -> ("Value"=w4995:dbl)  [unwired: 2 in, 2 out]
                n2594 = property on="Rise/Fall in points" class="DigNum (strict)"() -> ("Value"=w4996:i32)  [unwired: 2 in, 2 out]
                n2595 = property on="Number of Points per cycle" class="DigNum (strict)"() -> ("Value"=w4997:i32)  [unwired: 2 in, 2 out]
                n2596 = property on="Number of Cycles" class="DigNum (strict)"() -> ("Value"=w4998:dbl)  [unwired: 2 in, 2 out]
                n2597 = property on="Amplitude (Amps)" class="DigNum (strict)"() -> ("Value"=w4999:dbl)  [unwired: 2 in, 2 out]
                n2598 = property on="Offset (Amps)" class="DigNum (strict)"() -> ("Value"=w5000:dbl)  [unwired: 2 in, 2 out]
                n2599 = property on="Start Phase \n(Degrees)" class="DigNum (strict)"() -> ("Value"=w5001:dbl)  [unwired: 2 in, 2 out]
                n2600 = property on="Number of Points per cycle" class="DigNum (strict)"() -> ("Value"=w5002:i32)  [unwired: 2 in, 2 out]
                n2601 = property on="Number of Cycles" class="DigNum (strict)"() -> ("Value"=w5003:dbl)  [unwired: 2 in, 2 out]
                n2602 = Bundle(cluster=w4936, "Value"="High Current (Amps)", "Value"="Filter\nCount", "Value"=w4951, "Value"=w4952, "Value"="Low Current (Amps)", "Value"="Number of Readings", "Value"="Y Axis:", "Value"="Delay (mS) - settle time", "Value"="Voltage Measure Range", "Value"="DAMPING", "Value"="Measurement Integration (NPLCs)", "Value"="Current Source \nVoltage Compliance (V)", "Value"="X Axis:", "Value"="Current Source Range", "Value"="Start Current (Amps)", "Value"="Number of sweep points", "Value"="Start Voltage  (Volts)", "Value"="Stop Current (Amps)", "Value"=w5022, "Value"="Number of sweep points", "Value"=w5058, "Value"="Define source points with an:", "Value"="Delay (settle time in mS)", "Value"="Start Level", "Value"=w5021, "Value"="DIFF COND DAMPING", "Value"="Stop Level", "Value"="Number of steps", "Value"="Repeat Filter Count:", "Value"="Vertical Axis:", "Value"="Voltage Measure Range", "Value"=w5017, "Value"="Horizontal Axis:", "Value"="Current Source \nVoltage Compliance (V)", "Value"="Measurement Integration (NPLCs)", "Value"="Resistance in Ohms", "Value"="Stop Voltage (Volts)", "Value"="X Axis:", "Value"=w5019, "Value"="Number of Readings", "complete number of cycles"=w5023, "Value"=w5018, "Value"="Delay - pulse settle time in mS", "Value"="Stop Pulse Level (Amps)", "Value"="Pulse Level (Amps)", "Value"="Voltage Measure Range", "Value"="Start Pulse Level (Amps)", "Value"="Y Axis:", "Value"="Pulse Width (mS)", "Value"="Interval between Pulses (NPLC)", "Value"="Current Source \nVoltage Compliance (V)", "Value"="Sweep Type", "Value"=w5057, "Value"=w5020, "Value"=w5056, "Value"=w5055, "Value"=w5054, "Value"=w5053, "Value"=w5052, "Value"=w5051, "Value"=w5050, "Value"=w5049, "Value"=w5048, "Value"=w5047, "Value"=w5046, "Value"=w5045, "Value"=w5044, "Value"=w5043, "Value"="DEFAULT setup", "Value"=w5042, "result string"=w5041, "result string"=w5040, "result string"=w5039, "result string"=w5038, "result string"=w5037, "result string"=w5036, "Value"=w5029, "Value"=w5030, "Value"=w5035, "String"=w5034, "PULSE - SWEEP #STEPS"="Number of Pulses", "Sawtooth NUM CYCLES"=w4986, "Sawtooth Offset (Amps) 2"=w4987, "Duty Cycle (%) 2"=w4988, "Start Phase \n(Degrees) 2"=w4989, "SQUARE Number of Points per cycle 2"=w4990, "SQUARE Number of Cycles 2"=w4991, "SQUARE Amplitude (Amps) 2"=w4992, "SQUARE Offset (Amps) 2"=w4993, "SQUARE Duty Cycle (%) 3"=w4994, "SQUARE Start Phase \n(Degrees) 3"=w4995, "SQUARE Rise/Fall in points 2"=w4996, "SINE Number of Points per cycle 2"=w4997, "SINE Number of Cycles 2"=w4998, "SINE Amplitude (Amps) 2"=w4999, "SINE Offset (Amps) 2"=w5000, "SINE Start Phase \n(Degrees) 3"=w5001, "NOISE Number of Points per cycle 2"=w5002, "NOISE Number of Cycles 2"=w5003, "NOISE Standard Deviation 2"=w5004, "NOISE Offset (Amps) 2"=w5005, "Analog filter - \nTau in # points 2"=w5006, "ScratchPad Array 2"=w4883, "ScratchPad Array Cnt 2"=w4887, "Item Names"=w5016, "ADD 5"=w5015, "Complete Array 2"=w5014, "Complete Array Cnt 2"=w5013, "Item Names 5"=w5012, "ADD 7"=w5011, "waveform holder 2"=w5010, "ADD 6"=w5009, "ADD 8"=w5008, "ADD 9"=w5007, "Trace offset (% Pk-Pk): 2"="Trace offset (% Pk-Pk):", "phase enable 2"=w4984, "Phase Value 2"=w4983, "triggerline 2"=w4982, "Pulse Off Level (Amps) 2"="Pulse Off Level (Amps)", "ARB VOLT COMP"=w4981, "nV CAP"=w4912, "Pulse Filter"=w4966, "Pulse FIlter Count"="Pulse Filter Count", "Setup String"=w4914, "DCON filter state"=w4913, "Source Level (Amps) 3"=w4911, "Current Source \nVoltage Compliance (V) 4"=w4910, "Start Current (Amps) 3"=w4909, "Stop Current (Amps) 3"=w4908, "Number of sweep points 3"=w4907, "Sweep Type 3"=w4906, "Current Source \nVoltage Compliance (V) 5"=w4905, "Delay (settle time in sec) 3"=w4904, "enable measure 3"=w4903, "Voltage Measure Range 3"=w4902, "Measurement Integration \n(NPLCs) 3"=w4901, "Waveform Type  3"=w4900, "I Sweep V Measure Data 3"=w4899, "Ramp from: (Amps) 3"=w4898, "Ramp to: (Amps) 3"=w4897, "Duty Cycle (%) 4"=w4896, "Amplitude (Amps) 4"=w4895, "Offset (Amps) 4"=w4894, "Duty Cycle (%) 5"=w4893, "Amplitude (Amps) 5"=w4892, "Offset (Amps) 5"=w4891, "Signal Repetition \nFrequency (Hz) 3"=w4890, "Voltage\n Compliance3"=w4889, "Number of Zero Measurements 2"=w4888) -> (w4968:T10)
                "output cluster" <- w4968
                n2603 = property on="Default path" class="Path"() -> ("Value"=w4979:path)  [unwired: 2 in, 2 out]
                n2604 = Build Path(base path=w4979, name or relative path="DefaultTestFile.cfg" ("file path (dialog if empty)")) -> (appended path=w4978:path)
                n2605 = Flatten To String(anything=w4968) -> (data string=w5024:string)  [unwired: 3 in, 2 out]
                n2606 = Delete(path (use dialog)=w4978) -> (deleted path=w5026:path, error out=→"error out 5":errorcluster)  [unwired: 4 in, 1 out]
                n2607 = call "WriteToFile.vi"("character string"=w5024, "file path (dialog if empty)"=w5026) -> ("new file path (Not A Path if cancelled)"=w5025:path)  [unwired: 3 in]
                n2608 = Flatten To String(anything=w4968) -> (data string=w5028:string)  [unwired: 3 in, 2 out]
